vi "Migrate Installer To Current LabVIEW Version.vi"() -> ()   [LabVIEW 2013]
panel:
  out "error out":errorcluster
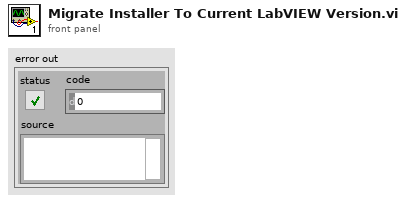
[diagram p1: front panel]
types:
  T1 = enum16{"open", "replace", "create", "open or create", "replace or create", "replace or create with confirmation"}
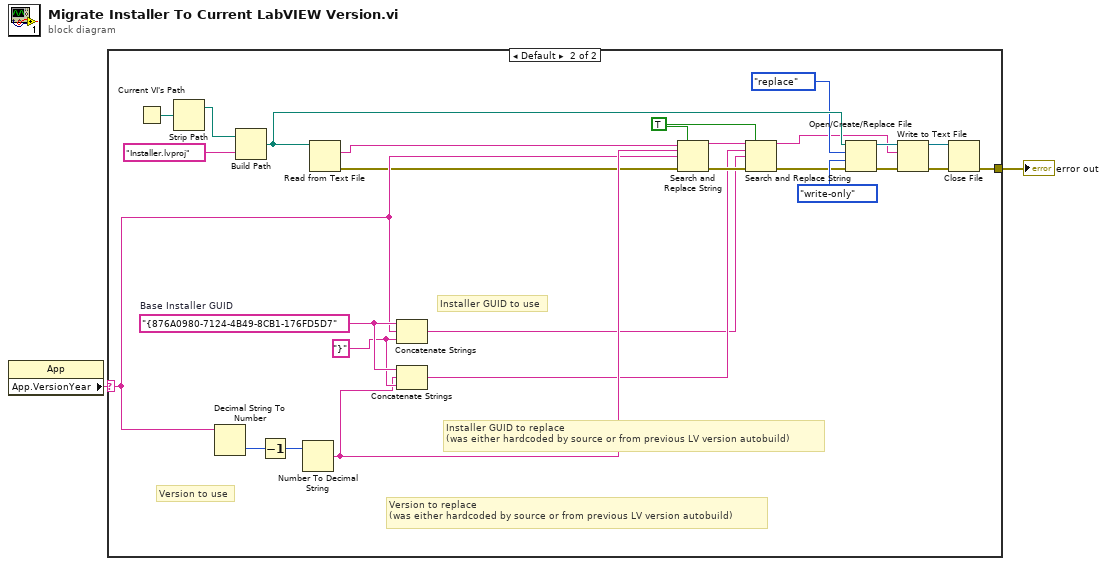
[diagram p0: block diagram]
diagram:
  n1 = property class="App"() -> ("App.VersionYear"=w2:string)  [unwired: 2 in, 2 out]
  n2 = case shown="Default" w2 {
    selector: w2 -> [_ w12]
    tunnel: [_ w3] -> w1
    frame "2013" {
      # "No updates needed. Project is saved with 2013 hard coded into it"
    }
    frame Default {
      w14 = "}"
      w15 = "{876A0980-7124-4B49-8CB1-176FD5D7"  # Base Installer GUID
      w4 = TRUE ("replace all? (F)")
      # "Version to use"
      # "Version to replace\n(was either hardcoded by source or from previous LV version autobuild)"
      # "Installer GUID to replace\n(was either hardcoded by source or from previous LV version autobuild)"
      # "Installer GUID to use"
      n3 = Current VI's Path() -> (path=w28:path)
      n4 = Strip Path(path=w28) -> (stripped path=w27:path)  [unwired: 1 out]
      n5 = Decimal String To Number(string=w12) -> (number=w17:i32)  [unwired: 2 in, 1 out]
      n6 = Build Path(base path=w27, name or relative path="Installer.lvproj") -> (appended path=w25:path)
      n7 = Decrement(x=w17) -> (x-1=w16:i32)
      n8 = Number To Decimal String(number=w16) -> (decimal integer string=w13:string)  [unwired: 1 in]
      n9 = Read from Text File(file (use dialog)=w25) -> (text=w10:string, error out=w11:errorcluster)  [unwired: 3 in, 2 out]
      n10 = Concatenate Strings(w15, w12, w14) -> (w5:string)
      n11 = Concatenate Strings(w15, w13, w14) -> (w6:string)
      n12 = Search and Replace String(replace all?=w4, input string=w10, search string=w13, replace string=w12, error in=w11) -> (result string=w8:string, error out=w19:errorcluster)  [unwired: 3 in, 2 out]
      n13 = Search and Replace String(replace all?=w4, input string=w8, search string=w6, replace string=w5, error in=w19) -> (result string=w7:string, error out=w9:errorcluster)  [unwired: 3 in, 2 out]
      n14 = Open/Create/Replace File(file path (use dialog)=w25, error in=w9, operation (0:open)=T1."replace", access (0:read/write)=enum16{"read/write", "read-only", "write-only"}."write-only") -> (refnum out=w22:refnum<file>, error out=w23:errorcluster)  [unwired: 2 in, 1 out]
      n15 = Write to Text File(file (use dialog)=w22, text=w7, error in=w23) -> (refnum out=w24:refnum<file>, error out=w18:errorcluster)  [unwired: 1 in, 1 out]
      n16 = Close File(refnum=w24, error in=w18) -> (error out=w3:errorcluster)  [unwired: 1 out]
    }
  }
  "error out" <- w1
